vi "ApplyLayoutFromUIarray.vi"(7 "Tbl Refnum":refnum<vi>, 8 "error in (no error)":errorcluster, 10 "ColLayout Array":T1[](array[typedef])) -> (0 "error out":errorcluster)   [LabVIEW 2013]
uses:
  TypeDefs/ColumnLayout_UI.ctl
  <vilib>/Utility/miscctls.llb/LVRowAndColumnTypeDef.ctl
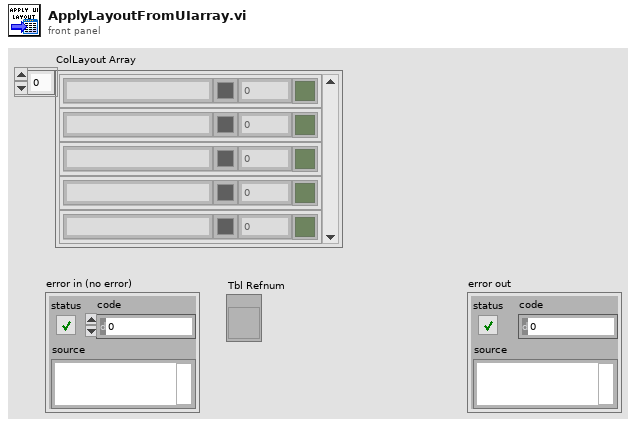
[diagram p1: front panel]
types:
  T1 = typedef "ColumnLayout_UI.ctl" = cluster{"Label":string, "Bgkd color":u32, "Width":u32, "Displayed?":bool}
  T2 = typedef "LVRowAndColumnTypeDef.ctl" = cluster{"Row":i32, "Column":i32}
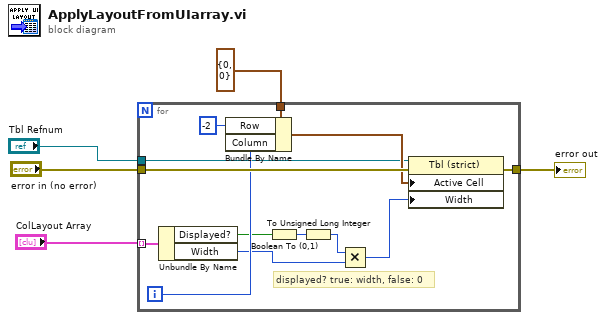
[diagram p0: block diagram]
diagram:
  n1 = for {
    tunnel: "error in (no error)" -> [w18]
    tunnel: [w17] -> w4
    tunnel: "ColLayout Array" -> [w13] mode=indexing
    tunnel: T2 {"Row"=0, "Column"=0} ("Active Cell:Active Cell") -> [w16]
    tunnel: "Tbl Refnum" -> [w11]
    i -> [w15]
    # "displayed? true: width, false: 0"
    n2 = Unbundle By Name(w13) -> ("Displayed?"=w8:bool, "Width"=w7:u32)
    n3 = Bundle By Name(cluster=w16, "Row"=-2, "Column"=w15) -> (w12:T2)
    n4 = Boolean To (0,1)(Boolean=w8) -> (0, 1=w10:i16)
    n5 = To Unsigned Long Integer(number=w10) -> (unsigned 32bit integer=w9:u32)
    n6 = Multiply(x=w9, y=w7) -> (x*y=w6:u32)
    n7 = property on="Property Node" class="Tbl (strict)"(reference=w11, error in=w18, "Active Cell"=w12, "Width"=w6) -> (error out=w17:errorcluster)  [unwired: 1 out]
  }
  "error out" <- w4
